vi "Read N channel.vi"(8 "error in (no error)":errorcluster, 11 "Master CR in":refnum<class "Master CR.lvclass">) -> (0 "error out":errorcluster, 2 "N channel":T1, 3 "Master CR out":refnum<class "Master CR.lvclass">)   [LabVIEW 2021, in "Master CR.lvclass"]
uses:
  Master CR.lvclass
  Modbus_v121c/Data Model/N channel.ctl
  Master CR.lvclass/Master CR.ctl
  Modbus_v121c/Data Model/Device Data Model.lvclass
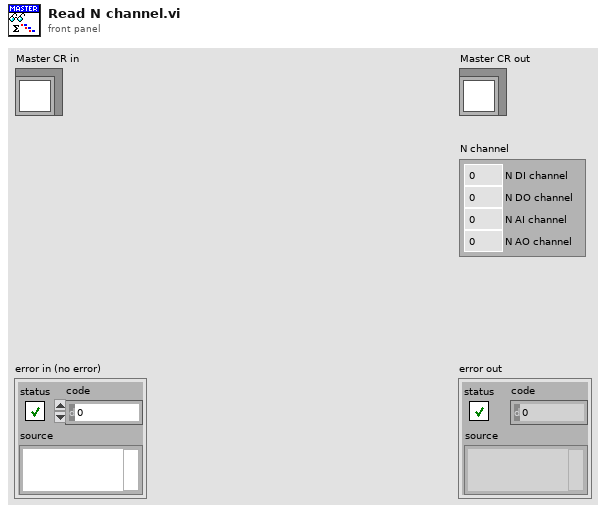
[diagram p1: front panel]
types:
  T1 = typedef "Device Data Model.lvclass/N channel.ctl" = cluster{"N DI channel":i32, "N DO channel":i32, "N AI channel":i32, "N AO channel":i32}
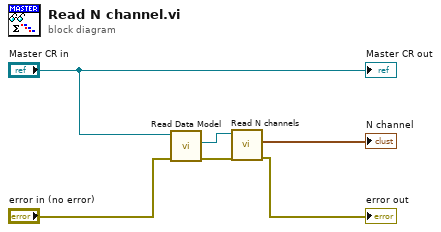
[diagram p0: block diagram]
diagram:
  n1 = call "Read Data Model.vi"("error in (no error)"="error in (no error)", "Master CR in"="Master CR in") -> ("error out"=w1:errorcluster, "Data Model"=w2:refnum<class "Device Data Model.lvclass">)  [unwired: 7 in, 1 out]
  n2 = call-dynamic "Read N channels.vi"("error in (no error)"=w1, "device data model in"=w2) -> ("error out"=→"error out":errorcluster, "N channel"=→"N channel":T1)  [unwired: 7 in, 1 out]
  "Master CR out" <- "Master CR in"
